vi "ReadDigitizerConfig(SubVI).vi"(8 "error in (no error)":errorcluster, 11 "appended path":path) -> (0 "error out":errorcluster, 3 "FLImDAQ":T1 {"trigger delay" format="%^#.4e"; "trigger level" min=0.0 max=3.5 step=0.5 format="%.2f"; "vertical offset" format="%.4f"; "vertical range" format="%.2f"; "min sample rate" format="%#.2p"})   [LabVIEW 2020]
uses:
  FLImDAQ.ctl
  <instrlib>/niScope/Controls/niScope trigger source.ctl
  <vilib>/Utility/file.llb/Read Delimited Spreadsheet (string).vi
  <vilib>/addons/_JKI.lib/Serialization/JSON/JKI JSON Serialization.lvlib
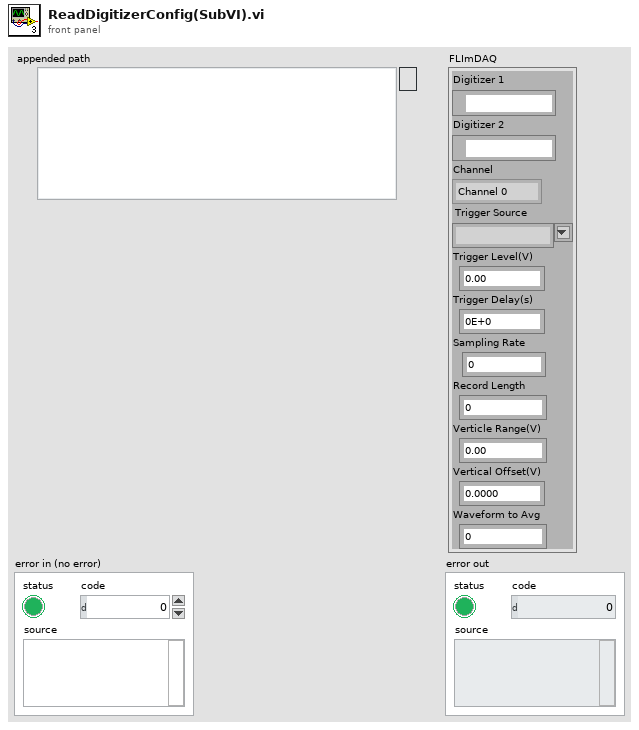
[diagram p1: front panel]
types:
  T1 = typedef "FLImDAQ.ctl" = cluster{"Digitizer 1":refnum<k15>, "Digitizer 2":refnum<k15>, "Channel":enum16{"Channel 0", "Channel 1", "Channel 0&1"}, "trigger source":T2, "trigger level":dbl, "trigger delay":dbl, "min sample rate":dbl, "min record length":i32, "vertical range":dbl, "vertical offset":dbl, "Waveform to Avg":i16}
  T2 = typedef "niScope trigger source.ctl" = string
  T3 = cluster{"Digitizer1":string, "Digitizer2":string, "Channel":enum16{"Channel 0", "Channel 1", "Channel 0&1"}, "trigger source":T2, "trigger level":dbl, "trigger delay":dbl, "min sample rate":dbl, "min record length":i32, "vertical range":dbl, "vertical offset":dbl, "Waveform to Avg":i32}
  T4 = cluster{"resource name":refnum<k15>, "resource name 2":refnum<k15>, "Channel":enum16{"Channel 0", "Channel 1", "Channel 0&1"}, "trigger source":T2, "trigger level":dbl, "trigger delay":dbl, "min sample rate":dbl, "min record length":i32, "vertical range":dbl, "vertical offset":dbl, "number of records":i32}
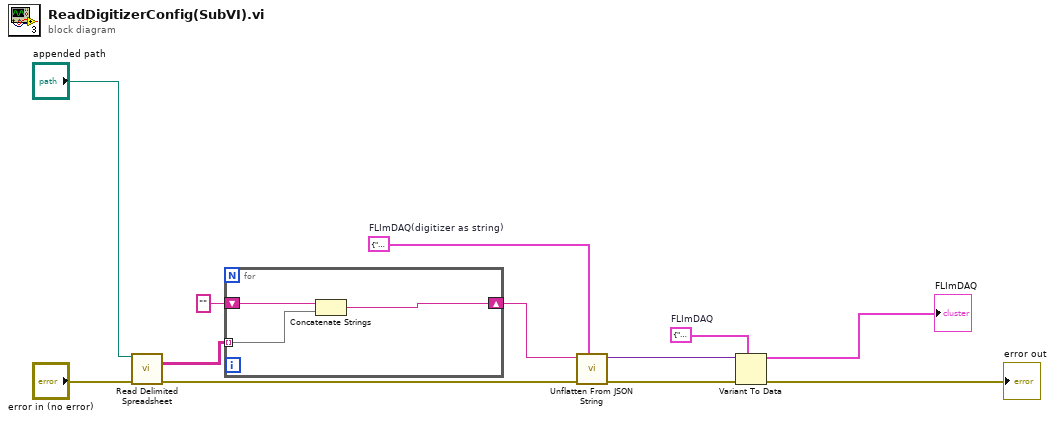
[diagram p0: block diagram]
diagram:
  w12 = T3 {"Digitizer1"="", "Digitizer2"="", "Channel"=enum."Channel 0", "trigger source"="VAL_EXTERNAL", "trigger level"=0.5, "trigger delay"=1.35e-07, "min sample rate"=12500000000.0, "min record length"=2500, "vertical range"=1.0, "vertical offset"=-0.25, "Waveform to Avg"=2000}  # FLImDAQ(digitizer as string)
  w11 = T4 {"resource name"="", "resource name 2"="", "Channel"=enum."Channel 0", "trigger source"="VAL_EXTERNAL", "trigger level"=0.5, "trigger delay"=1.35e-07, "min sample rate"=12500000000.0, "min record length"=2500, "vertical range"=1.0, "vertical offset"=-0.25, "number of records"=2000}  # FLImDAQ
  n1 = call-poly <vilib>:"Read Delimited Spreadsheet.vi"("file path (dialog if empty)"="appended path", "error in (no error)"="error in (no error)") -> ("all rows"=w2:string[][], "error out"=w7:errorcluster)  [unwired: 8 in, 4 out]
  n2 = for {
    tunnel: w2 -> [w15] mode=indexing
    shift-right: [w13] -> w5
    shift-left: "" -> [w14]
    n3 = Concatenate Strings(w14, w15) -> (w13:string)
  }
  n4 = call <vilib>:"Unflatten From JSON String.vi"("Type and Defaults"=w12, "error in"=w7, "JSON String"=w5) -> ("error out"=w8:errorcluster, "Variant"=w4:variant)  [unwired: 7 in]
  n5 = Variant To Data(error in=w8, type=w11, Variant=w4) -> (data=→"FLImDAQ":T4, error out=→"error out":errorcluster)
